vi "Translate_BOOLEAN.vi"(8 "error IN":errorcluster, 10 "Cle":string, 11 "Bool Refnum":refnum<vi>) -> (0 "error out":errorcluster)   [LabVIEW 2013]
uses:
  Dictionnary/EnumCommandDictionnaire.ctl
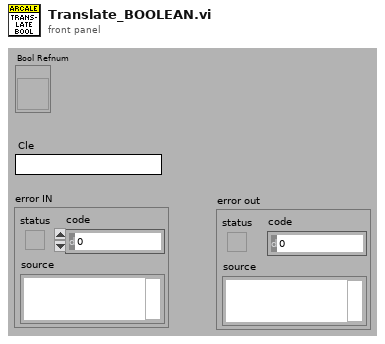
[diagram p1: front panel]
types:
  T1 = typedef "EnumCommandDictionnaire.ctl" = enum16{"Load", "Translate", "Save", "GetDico", "Set : A traduire = Vrai", "Set : A Traduire = Faux", "SetDico"}
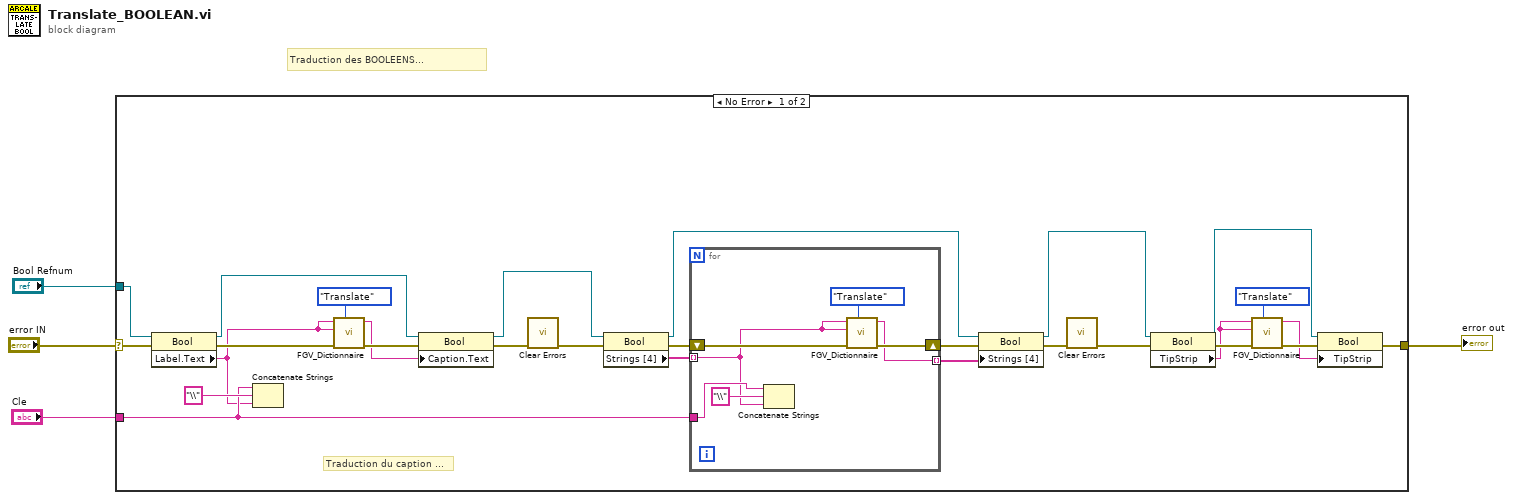
[diagram p0: block diagram]
diagram:
  # "Traduction des BOOLEENS..."
  n1 = case shown="No Error" "error IN" {
    selector: "error IN" -> [w32 w40]
    tunnel: "Bool Refnum" -> [w31 _]
    tunnel: "Cle" -> [w24 _]
    tunnel: [w11 w40] -> w1
    frame No Error {
      # "Traduction du caption ..."
      n2 = property class="Bool"(reference=w31, error in=w32) -> (reference out=w29:refnum<vi>, error out=w19:errorcluster, "Label.Text"=w14:string)
      n3 = Concatenate Strings(w24, "\\" ("string"), w14) -> ()  [unwired: 1 out]
      n4 = call "FGV_Dictionnaire.vi"("Command"=EnumCommandDictionnaire."Translate", "error in (no error)"=w19, "Chaîne"=w14, "Clé"=w14) -> ("error out"=w18:errorcluster, "Traduction"=w17:string)  [unwired: 5 in, 1 out]
      n5 = property class="Bool"(reference=w29, error in=w18, "Caption.Text"=w17) -> (reference out=w28:refnum<vi>, error out=w27:errorcluster)
      n6 = call <vilib>:"Clear Errors.vi"("error in (no error)"=w27) -> ("error out"=w15:errorcluster)  [unwired: 6 in]
      n7 = property class="Bool"(reference=w28, error in=w15) -> (reference out=w22:refnum<vi>, error out=w25:errorcluster, "Strings [4]"=w26:string[])
      n8 = for {
        tunnel: w26 -> [w33] mode=indexing
        shift-right: [w35] -> w23
        shift-left: w25 -> [w36]
        tunnel: w24 -> [w38]
        tunnel: [w34] -> w16 mode=indexing
        n9 = Concatenate Strings(w38, "\\" ("string"), w33) -> ()  [unwired: 1 out]
        n10 = call "FGV_Dictionnaire.vi"("Command"=EnumCommandDictionnaire."Translate", "error in (no error)"=w36, "Chaîne"=w33, "Clé"=w33) -> ("error out"=w35:errorcluster, "Traduction"=w34:string)  [unwired: 5 in, 1 out]
      }
      n11 = property class="Bool"(reference=w22, error in=w23, "Strings [4]"=w16) -> (reference out=w12:refnum<vi>, error out=w21:errorcluster)
      n12 = call <vilib>:"Clear Errors.vi"("error in (no error)"=w21) -> ("error out"=w13:errorcluster)  [unwired: 6 in]
      n13 = property class="Bool"(reference=w12, error in=w13) -> (reference out=w10:refnum<vi>, error out=w8:errorcluster, "TipStrip"=w6:string)
      n14 = call "FGV_Dictionnaire.vi"("Command"=EnumCommandDictionnaire."Translate", "error in (no error)"=w8, "Chaîne"=w6, "Clé"=w6) -> ("error out"=w7:errorcluster, "Traduction"=w5:string)  [unwired: 5 in, 1 out]
      n15 = property class="Bool"(reference=w10, error in=w7, "TipStrip"=w5) -> (error out=w11:errorcluster)  [unwired: 1 out]
    }
    frame Error {
    }
  }
  "error out" <- w1
